vi "Get Service Descriptor.vi"(8 "error in":errorcluster) -> (0 "error out":errorcluster, 3 "service descriptor":T1)   [LabVIEW 2022 SP3, in "Crosstalk_Class D Amplifier.lvlib"]
uses:
  Crosstalk_Class D Amplifier.lvlib
  <vilib>/Plug-In SDKs/Measurements/Helpers/TypeDefs/Service Descriptor.ctl
  <vilib>/Plug-In SDKs/Measurements/Helpers/TypeDefs/Measurement Details.ctl
  <vilib>/Plug-In SDKs/Measurements/Helpers/TypeDefs/Measurement Annotation.ctl
  <vilib>/Plug-In SDKs/Measurements/NI Measurement Plug-In SDK.lvlib
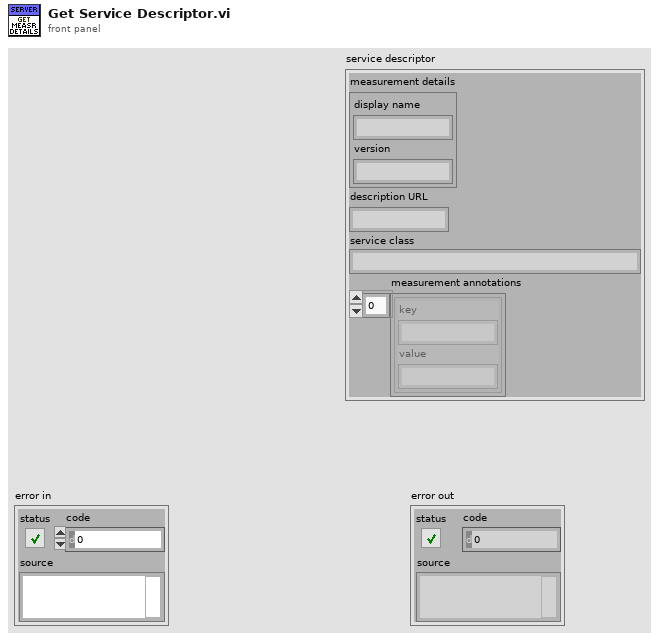
[diagram p1: front panel]
types:
  T1 = typedef "NI Measurement Plug-In SDK.lvlib/Service Descriptor.ctl" = cluster{"measurement details":T2, "description URL":string, "service class":string, "measurement annotations":T3[]}
  T2 = typedef "NI Measurement Plug-In SDK.lvlib/Measurement Details.ctl" = cluster{"display name":string, "version":string}
  T3 = typedef "NI Measurement Plug-In SDK.lvlib/Measurement Annotation.ctl" = cluster{"key":string, "value":string}
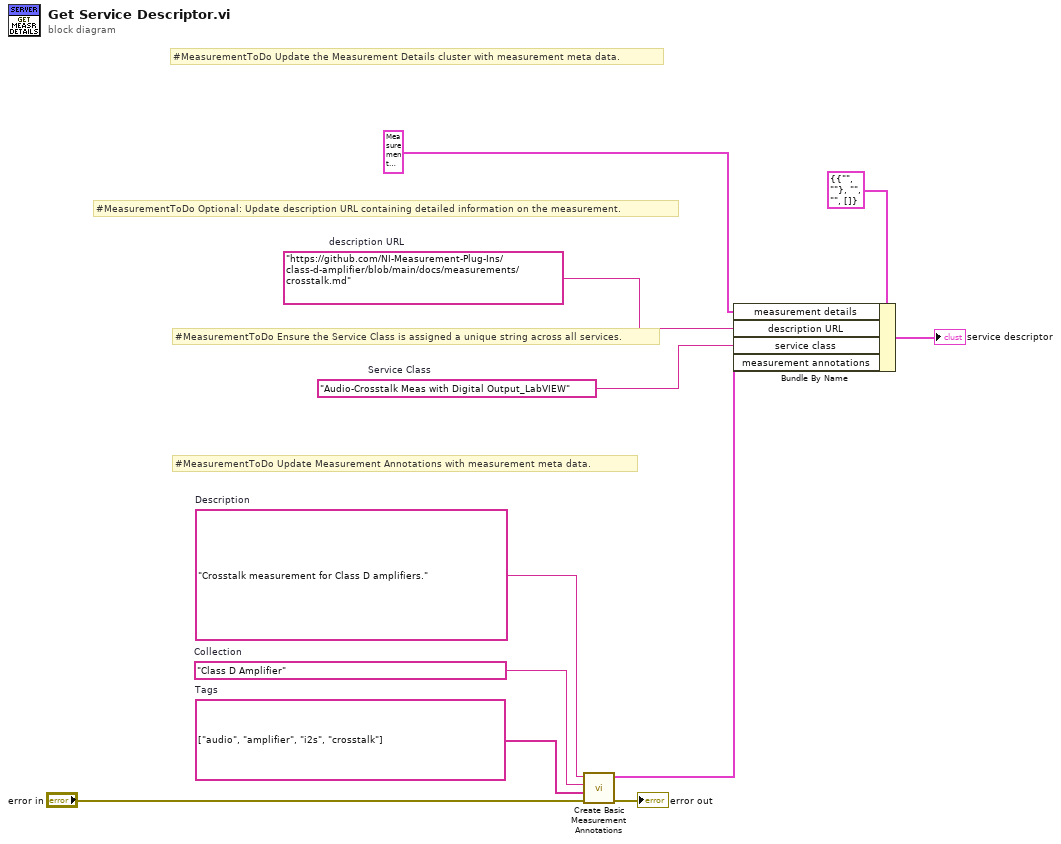
[diagram p0: block diagram]
diagram:
  w4 = "https://github.com/NI-Measurement-Plug-Ins/class-d-amplifier/blob/main/docs/measurements/crosstalk.md"  # description URL
  w7 = string[] ["audio", "amplifier", "i2s", "crosstalk"]  # Tags
  w8 = "Class D Amplifier"  # Collection
  w9 = "Crosstalk measurement for Class D amplifiers."  # Description
  w2 = "Audio-Crosstalk Meas with Digital Output_LabVIEW"  # Service Class
  # "#MeasurementToDo Optional: Update description URL containing detailed information on the measurement."
  # "#MeasurementToDo Update Measurement Annotations with measurement meta data."
  # "#MeasurementToDo Ensure the Service Class is assigned a unique string across all services."
  # "#MeasurementToDo Update the Measurement Details cluster with measurement meta data."
  n1 = call <vilib>:"Create Basic Measurement Annotations.vi"("error in"="error in", "tags"=w7, "collection"=w8, "description"=w9) -> ("error out"=→"error out":errorcluster, "measurement annotations"=w1:T3[])  [unwired: 6 in]
  n2 = Bundle By Name(cluster=T1 {"measurement details"={"display name"="", "version"=""}, "description URL"="", "service class"="", "measurement annotations"=[]} ("service descriptor"), "measurement details"=T2 {"display name"="Crosstalk", "version"="1.0.0"} ("Measurement Details"), "description URL"=w4, "service class"=w2, "measurement annotations"=w1) -> (→"service descriptor":T1)
